vi "22_09_ex_02.vi"() -> ()   [LabVIEW 2025]
uses:
  Control 1.ctl
panel:
  out "Array 2":bool[][](array[boolean])
  in  "Array":dbl[][](array[numeric])
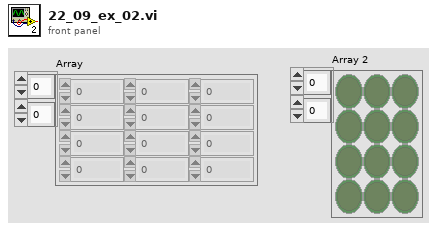
[diagram p1: front panel]
types:
  T1 = typedef "Control 1.ctl" = void[]
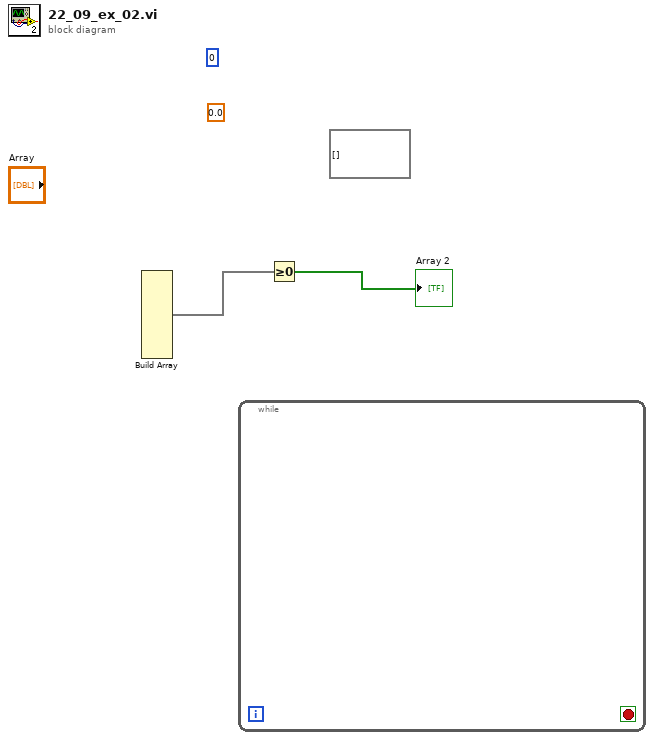
[diagram p0: block diagram]
diagram:
  (unwired) T1 []
  (unwired) 0.0
  (unwired) 0
  n1 = Build Array() -> (w2:void[])  [unwired: 11 in]
  n2 = while {
    stop <- _ stop-if-true
  }
  n3 = Greater Or Equal To 0?(x=w2) -> (x >= 0?=→"Array 2":bool[])
